vi "TurnAndZeroRTv2.vi"   [LabVIEW 2015]
types:
  T1 = typedef "WPI_MotorControlDeviceRef.ctl" = cluster{"DeviceStatus":errorcluster, "Type":T2, "PWM":cluster{"PWM Channel":T3, "DeadBand":T4}, "CAN":cluster{"Device Number":u8, "Control Mode":T5, "Semaphore":T6, "Max Vout":dbl, "TalonSRX Control Mode":T7}, "Invert":bool}
  T2 = typedef "WPI_MotorControlType.ctl" = enum16{"PWM", "CAN", "CANTalonSRX"}
  T3 = typedef "FPGA_DIOPWMChannel.ctl" = enum8{"PWM 0", "PWM 1", "PWM 2", "PWM 3", "PWM 4", "PWM 5", "PWM 6", "PWM 7", "PWM 8", "PWM 9", "PWM MXP 0", "PWM MXP 1", "PWM MXP 2", "PWM MXP 3", "PWM MXP 4", "PWM MXP 5", "PWM MXP 6", "PWM MXP 7", "PWM MXP 8", "PWM MXP 9", "Invalid"}
  T4 = typedef "WPI_PWMDeadband.ctl" = cluster{"Name":string, "maxPositivePwm":i32, "minPositivePwm":i32, "centerPwm":i32, "maxNegativePwm":i32, "minNegativePwm":i32, "angularRange":u16}
  T5 = typedef "WPI_CANJaguar_ControlMode.ctl" = enum8{"Percent VBus", "Current", "Speed", "Position", "Voltage"}
  T6 = typedef "Semaphore RefNum" = refnum<k1>
  T7 = typedef "WPI_CANTalonSRX_APIControlMode.ctl" = enum8{"Percent VBus", "Speed", "Position", "Slave", "Unchanged / Invalid", "Voltage Compensation", "Current", "Motion Profile"}
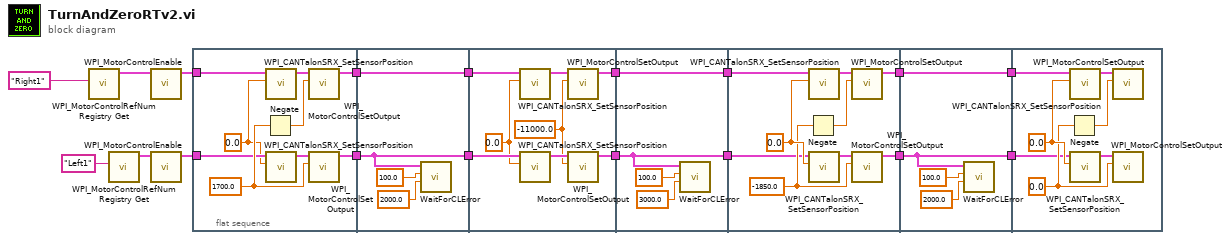
[diagram p0: block diagram]
diagram:
  n1 = call <vilib>:"WPI_MotorControlRefNum Registry Get.vi"("refnum name"="Right1") -> ("MotorControlDevRef"=w3:T1)  [unwired: 9 in, 1 out]
  n2 = call <vilib>:"WPI_MotorControlRefNum Registry Get.vi"("refnum name"="Left1") -> ("MotorControlDevRef"=w5:T1)  [unwired: 9 in, 1 out]
  n3 = call <vilib>:"WPI_MotorControlEnable.vi"("CAN MotorDevRef"=w3) -> ("CAN MotorDevRef"=w4:T1)  [unwired: 9 in, 1 out]
  n4 = call <vilib>:"WPI_MotorControlEnable.vi"("CAN MotorDevRef"=w5) -> ("CAN MotorDevRef"=w6:T1)  [unwired: 9 in, 1 out]
  n5 = flat-sequence {
    tunnel: w6 -> [w23]
    tunnel: w4 -> [w21]
    tunnel: [w25] -> w18
    tunnel: [w24] -> w17
    tunnel: [w31] -> w16
    tunnel: w18 -> [w31]
    tunnel: [w28] -> w15
    tunnel: w17 -> [w28]
    tunnel: w16 -> [w39]
    tunnel: w15 -> [w38]
    tunnel: [w33] -> w14
    tunnel: [w32] -> w13
    tunnel: w14 -> [w43]
    tunnel: [w43] -> w12
    tunnel: w13 -> [w40]
    tunnel: [w40] -> w11
    tunnel: w12 -> [w48]
    tunnel: w11 -> [w47]
    tunnel: [w45] -> w10
    tunnel: [w44] -> w9
    tunnel: w10 -> [w56]
    tunnel: [w56] -> w8
    tunnel: w9 -> [w53]
    tunnel: [w53] -> w7
    tunnel: w7 -> [w57]
    tunnel: w8 -> [w58]
    frame #0 {
      w19 = 0.0 ("New Sensor Position")
      w27 = 1700.0
      n6 = Negate(x=w27) -> (-x=w26:dbl)
      n7 = call <vilib>:"WPI_CANTalonSRX_SetSensorPosition.vi"("New Sensor Position"=w19, "CAN Talon SRX Ref"=w21) -> ("CAN Talon SRX Ref"=w20:T1)  [unwired: 8 in, 1 out]
      n8 = call <vilib>:"WPI_CANTalonSRX_SetSensorPosition.vi"("New Sensor Position"=w19, "CAN Talon SRX Ref"=w23) -> ("CAN Talon SRX Ref"=w22:T1)  [unwired: 8 in, 1 out]
      n9 = call <vilib>:"WPI_MotorControlSetOutput.vi"("Output"=w26, "MotorControlDevRef"=w20) -> ("MotorControlDevRef"=w25:T1)  [unwired: 7 in, 2 out]
      n10 = call <vilib>:"WPI_MotorControlSetOutput.vi"("Output"=w27, "MotorControlDevRef"=w22) -> ("MotorControlDevRef"=w24:T1)  [unwired: 7 in, 2 out]
    }
    frame #1 {
      n11 = call "WaitForCLError.vi"("Timeout (ms)"=2000.0, "AllowedError"=100.0, "CAN Talon SRX Ref"=w28) -> ()  [unwired: 8 in, 1 out]
    }
    frame #2 {
      w34 = -11000.0 ("Output")
      w37 = 0.0 ("New Sensor Position")
      n12 = call <vilib>:"WPI_CANTalonSRX_SetSensorPosition.vi"("New Sensor Position"=w37, "CAN Talon SRX Ref"=w39) -> ("CAN Talon SRX Ref"=w36:T1)  [unwired: 8 in, 1 out]
      n13 = call <vilib>:"WPI_CANTalonSRX_SetSensorPosition.vi"("New Sensor Position"=w37, "CAN Talon SRX Ref"=w38) -> ("CAN Talon SRX Ref"=w35:T1)  [unwired: 8 in, 1 out]
      n14 = call <vilib>:"WPI_MotorControlSetOutput.vi"("Output"=w34, "MotorControlDevRef"=w36) -> ("MotorControlDevRef"=w33:T1)  [unwired: 7 in, 2 out]
      n15 = call <vilib>:"WPI_MotorControlSetOutput.vi"("Output"=w34, "MotorControlDevRef"=w35) -> ("MotorControlDevRef"=w32:T1)  [unwired: 7 in, 2 out]
    }
    frame #3 {
      n16 = call "WaitForCLError.vi"("Timeout (ms)"=3000.0, "AllowedError"=100.0, "CAN Talon SRX Ref"=w40) -> ()  [unwired: 8 in, 1 out]
    }
    frame #4 {
      w49 = -1850.0 ("Output")
      w52 = 0.0 ("New Sensor Position")
      n17 = Negate(x=w49) -> (-x=w46:dbl)
      n18 = call <vilib>:"WPI_CANTalonSRX_SetSensorPosition.vi"("New Sensor Position"=w52, "CAN Talon SRX Ref"=w48) -> ("CAN Talon SRX Ref"=w51:T1)  [unwired: 8 in, 1 out]
      n19 = call <vilib>:"WPI_CANTalonSRX_SetSensorPosition.vi"("New Sensor Position"=w52, "CAN Talon SRX Ref"=w47) -> ("CAN Talon SRX Ref"=w50:T1)  [unwired: 8 in, 1 out]
      n20 = call <vilib>:"WPI_MotorControlSetOutput.vi"("Output"=w46, "MotorControlDevRef"=w51) -> ("MotorControlDevRef"=w45:T1)  [unwired: 7 in, 2 out]
      n21 = call <vilib>:"WPI_MotorControlSetOutput.vi"("Output"=w49, "MotorControlDevRef"=w50) -> ("MotorControlDevRef"=w44:T1)  [unwired: 7 in, 2 out]
    }
    frame #5 {
      n22 = call "WaitForCLError.vi"("Timeout (ms)"=2000.0, "AllowedError"=100.0, "CAN Talon SRX Ref"=w53) -> ()  [unwired: 8 in, 1 out]
    }
    frame #6 {
      w60 = 0.0 ("Output")
      w63 = 0.0 ("New Sensor Position")
      n23 = Negate(x=w60) -> (-x=w59:dbl)
      n24 = call <vilib>:"WPI_CANTalonSRX_SetSensorPosition.vi"("New Sensor Position"=w63, "CAN Talon SRX Ref"=w58) -> ("CAN Talon SRX Ref"=w62:T1)  [unwired: 8 in, 1 out]
      n25 = call <vilib>:"WPI_CANTalonSRX_SetSensorPosition.vi"("New Sensor Position"=w63, "CAN Talon SRX Ref"=w57) -> ("CAN Talon SRX Ref"=w61:T1)  [unwired: 8 in, 1 out]
      n26 = call <vilib>:"WPI_MotorControlSetOutput.vi"("Output"=w59, "MotorControlDevRef"=w62) -> ()  [unwired: 7 in, 3 out]
      n27 = call <vilib>:"WPI_MotorControlSetOutput.vi"("Output"=w60, "MotorControlDevRef"=w61) -> ()  [unwired: 7 in, 3 out]
    }
  }
